vi "que_enqueue_message.vi"   [LabVIEW 2013]
doc: "For a regular message, enqueue the message. For a priority message, enqueue it at the front of the queue."
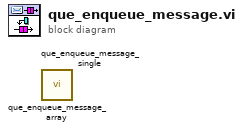
[diagram p0: block diagram]
diagram:
  n1 = call "que_enqueue_message_array.vi"() -> ()  [unwired: 10 in, 2 out]
  n2 = call "que_enqueue_message_single.vi"() -> ()  [unwired: 10 in, 2 out]
